vi "Configure Power Sensor Attenuation.vi"(7 "Attenuation (0.0)":dbl format="%^.3e", 8 "error in (no error)":errorcluster, 9 "State (Off)":bool, 10 "Instance (1)":i32=1 format="%.0g", 11 "VISA resource name":refnum<visa-resource-name>) -> (0 "error out":errorcluster, 3 "VISA resource name out":refnum<visa-resource-name>)   [LabVIEW 2015, in "Rohde&Schwarz CMXP GPRF.lvlib"]
doc: "Specifies external sensor attenuation settings.\n\nAttributes:\nRSCMXPGPRF_ATTR_SENSOR_MEASUREMENT_ATTENUATION_STATE\nRSCMXPGPRF_ATTR_SENSOR_MEASUREMENT_ATTENUATION\n\nRemote-control commands:\nCONFigure:GPRF:MEAS<i>:EPSensor:ATTenuation:STATe\nCONFigure:GPRF:MEAS<i>:EPSensor:ATTenuation"
uses:
  <instrlib>/Rohde&Schwarz CMXP GPRF/Rohde&Schwarz CMXP GPRF.lvlib
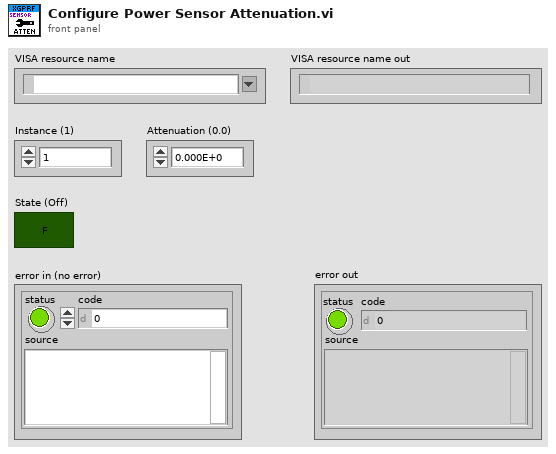
[diagram p1: front panel]
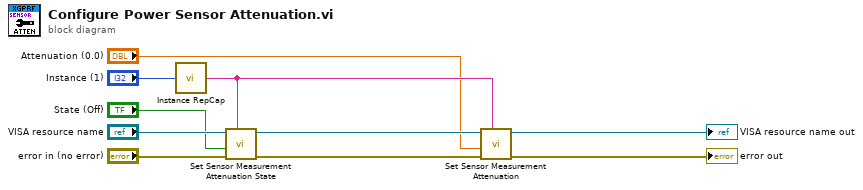
[diagram p0: block diagram]
diagram:
  n1 = call <instrlib>:"Instance RepCap.vi"("instance  in"="Instance (1)") -> ("instance out"=w3:string)
  n2 = call "Set Sensor Measurement Attenuation State"("Repeated Capabilities"=w3, "error in (no error)"="error in (no error)", "Sensor Measurement Attenuation State (OFF)"="State (Off)", "instrument handle"="VISA resource name") -> ("error out"=w8:errorcluster, "instrument handle out"=w7:refnum<visa-resource-name>)  [unwired: 6 in]
  n3 = call "Set Sensor Measurement Attenuation"("Repeated Capabilities"=w3, "error in (no error)"=w8, "Sensor Measurement Attenuation (0.0)"="Attenuation (0.0)", "instrument handle"=w7) -> ("error out"=→"error out":errorcluster, "instrument handle out"=→"VISA resource name out":refnum<visa-resource-name>)  [unwired: 6 in]
